vi "DSF Transfer Group.Sort by Priority.vi"(8 "error in (no error)":errorcluster, 11 "Transfer Groups":refnum<class "Transfer Group.lvclass">[](array[class])) -> (0 "error out":errorcluster, 3 "sorted Transfer Groups":refnum<class "Transfer Group.lvclass">[](array[class]))   [LabVIEW 2017, in "DSF.Engine.lvlib" / "Transfer Group.lvclass"]
uses:
  Transfer Group.lvclass
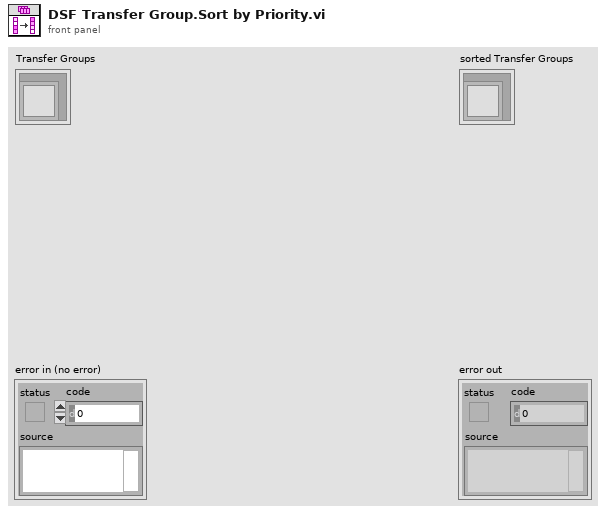
[diagram p1: front panel]
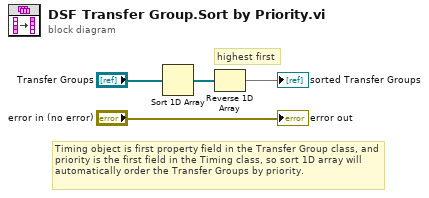
[diagram p0: block diagram]
diagram:
  # "highest first"
  # "Timing object is first property field in the Transfer Group class, and priority is the first field in the Timing class, so sort 1D array will automatically order the Transfer Groups by priority."
  n1 = Sort 1D Array(array="Transfer Groups") -> (sorted array=w3:refnum<class "Transfer Group.lvclass">[])
  n2 = Reverse 1D Array(array=w3) -> (reversed array=→"sorted Transfer Groups":refnum<class "Transfer Group.lvclass">[])
  "error out" <- "error in (no error)"
